vi "Auto.vi"() -> ()   [LabVIEW 2020]
uses:
  Global_Variable/Global.vi
  Global_Variable/A180648.vi
  Global_Variable/System_Conf.vi
  Libraries/S7/S7.lvlib
panel:
  out "前序":string
  out "用户事件输出":refnum<user-event>
  out "磨合正向初始化":bool
  out "工位三开始计时1":bool
  out "产品变更_Event":refnum<user-event>
  out "NVH":bool=TRUE
  out "T1+T2":dbl
  out "T2":dbl
  out "T1":dbl
  out "吸收电流":sgl
  out "输出扭矩(大)":sgl
  out "输入扭矩":sgl
  out "力特性逆向去程":bool
  out "力特性正向去程":bool
  out "力特性逆向回程":bool
  out "力特性正向回程":bool
  out "工位三开始计时":bool
  out "工位二开始计时":bool
  out "功能正向初始化":bool
  out "功能逆向初始化":bool
  out "空载逆向初始化":bool
  out "空载正向初始化":bool
  out "试验项目":T1(tab)
  out "拉力曲线":cluster{dbl[], dbl[]}[](graph)
  out "侧铆曲线":cluster{dbl[], dbl[]}[](graph)
  out "0°曲线":cluster{dbl[], dbl[]}[](graph)
  out "45°曲线":cluster{dbl[], dbl[]}[](graph)
  out "力特性试验":cluster{dbl[], dbl[]}[](graph)
  out "功能试验":cluster{dbl[], dbl[]}[](graph)
  out "电流特性试验":cluster{dbl[], dbl[]}[](graph)
  out "逆向空载试验":cluster{dbl[], dbl[]}[](graph)
  out "磨合":cluster{dbl[], dbl[]}[](graph)
  in  "判定结果":bool[][](array[boolean])=[[TRUE]]
  in  "STEP":string
  # "车速0"
  # "车速1"
  # "车速2"
  # "车速3"
  # "车速4"
  # "车速5"
  # "车速0"
  # "车速1"
  # "车速2"
  # "车速3"
  # "车速4"
  # "车速5"
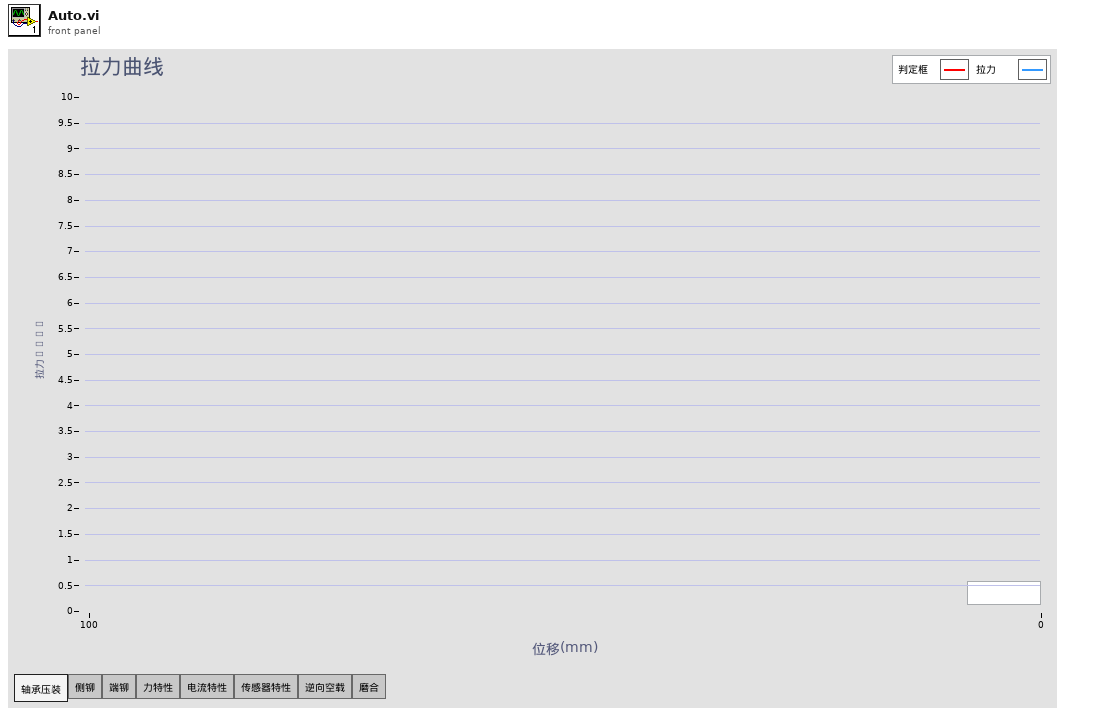
[diagram p1: front panel]
types:
  T1 = enum32{"轴承压装", "侧铆", "端铆", "力特性", "电流特性", "传感器特性", "逆向空载", "磨合"}
  T2 = enum32{"Invalid", "Standard", "Closed", "Hidden", "Minimized", "Maximized"}
  T3 = cluster{"输入轴扭矩":dbl, "输出轴扭矩小量程":dbl, "输出轴扭矩大量程":dbl}
  T4 = typedef "System_conf.ctl" = cluster{"空载滤波":bool, "逆向空载滤波":bool, "空载扭矩系数":dbl, "逆向空载扭矩系数":dbl}
  T5 = cluster{"1位移":cluster{"单位":string, "下限":dbl, "上限":dbl}, "1压力":cluster{"单位":string, "下限":dbl, "上限":dbl}}
  T6 = cluster{"第一段位移区间最大压力":cluster{"单位":string, "下限":dbl, "上限":dbl}, "第一段位移区间最小压力":cluster{"单位":string, "下限":dbl, "上限":dbl}, "压装最终位移":cluster{"单位":string, "下限":dbl, "上限":dbl}}
  T7 = cluster{"卡簧判定结果":cluster{"单位":string, "下限":dbl, "上限":dbl}}
  T8 = typedef "lveventtype.ctl" = enum32{"Null", "Timeout", "Annotation Menu Selection", "Annotation Menu Selection?", "App Instance Close", "App Instance Close?", "Autoscale Range Change", "Bookmark Info Change", "Cell Edit", "Cell Edit?", "Cursor Grab", "Cursor Grab?", "Cursor Menu Selection", "Cursor Menu Selection?", "Cursor Move", "Cursor Release", "Data Change", "Direction Change", "Display State Change", "Drag Ended", "Drag Enter", "Drag Leave", "Drag Over", "Drag Source Update", "Drag Starting", "Drag Starting?", "Drop", "Exec State Change", "Key Down", "Key Down?", "Key Repeat", "Key Repeat?", "Key Up", "Listbox Double Click", "Menu Activation?", "Menu Selection (App)", "Menu Selection? (App)", "Menu Selection (User)", "Mouse Down", "Mouse Down?", "Mouse Enter", "Mouse Leave", "Mouse Move", "Mouse Up", "Mouse Wheel", "NI Security User Change (App)", "Pane Size", "Panel Close", "Panel Close?", "Panel Resize", "Plot Attribute Change", "Scale Range Change", "Shortcut Menu Activation?", "Shortcut Menu Selection (App)", "Shortcut Menu Selection? (App)", "Shortcut Menu Selection (User)", "Tree Double Click", "Tree Drag", "Tree Drag?", "Tree Drop", "Tree Drop?", "Tree Item Close", "Tree Item Close?", "Tree Item Open", "Tree Item Open?", "User Event", "Value Change"}
  T9 = typedef "LVPoint32TypeDef.ctl" = cluster{"Horizontal":i32, "Vertical":i32}
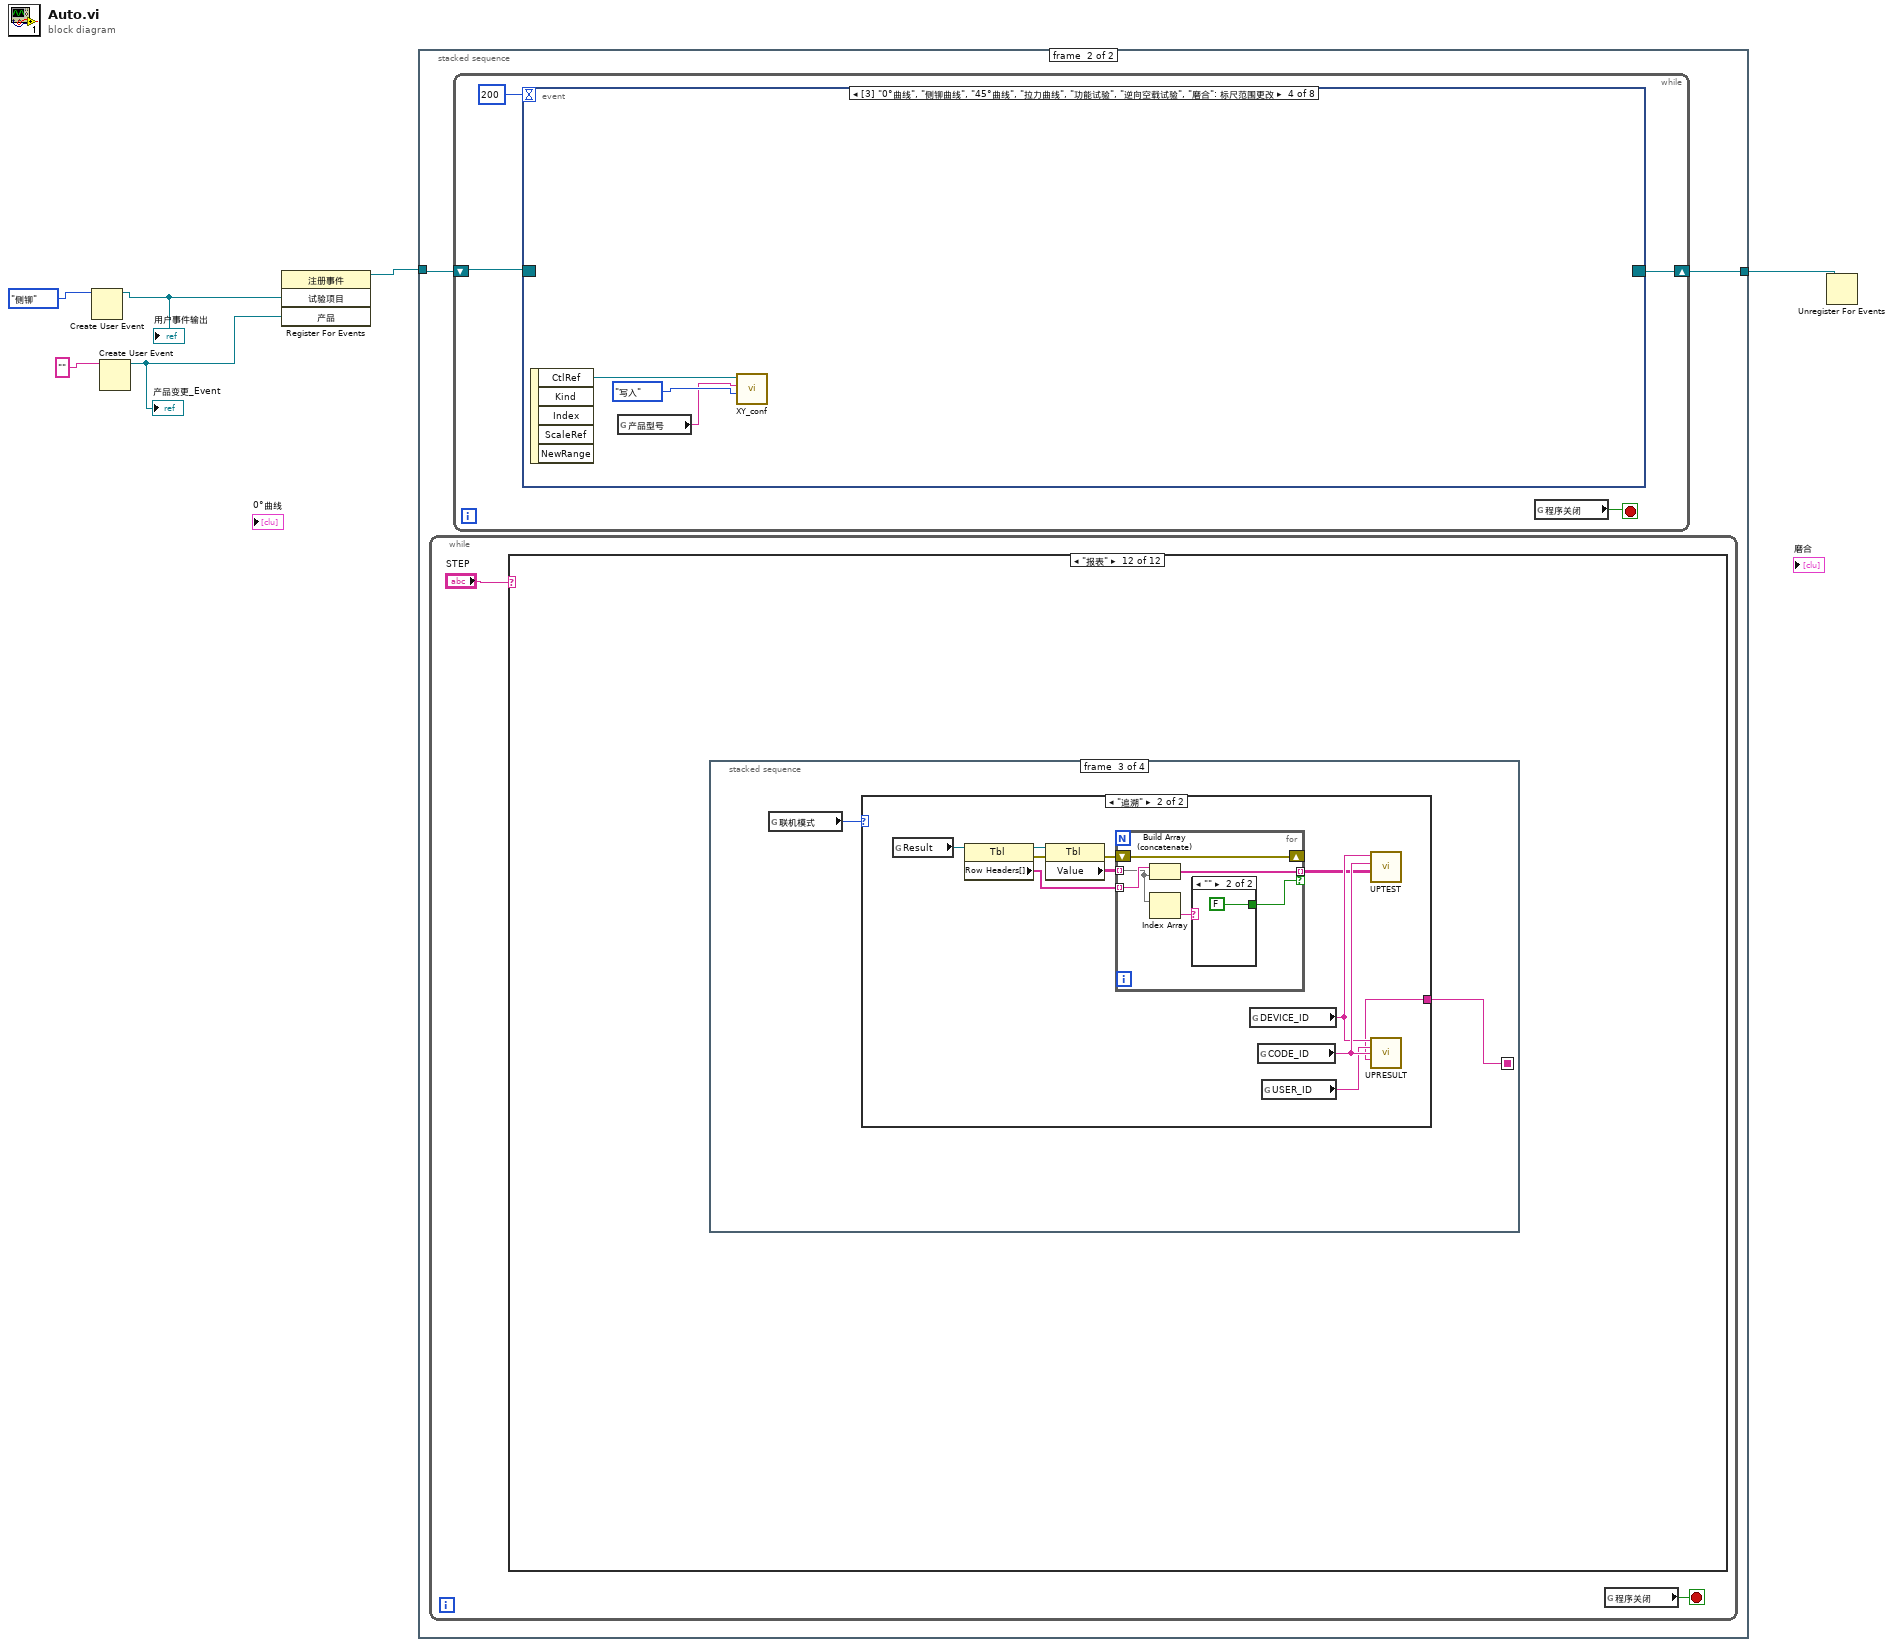
[diagram p0: block diagram]
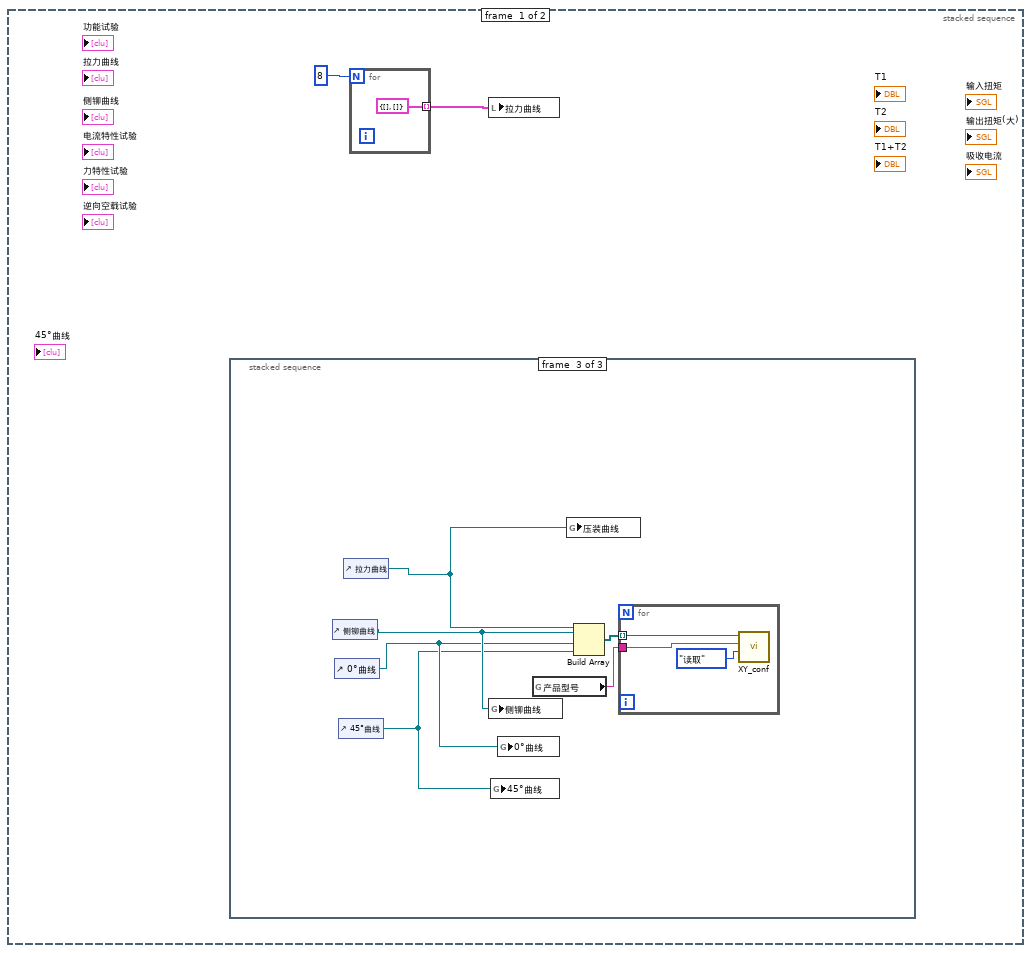
[diagram p2: hidden frame]
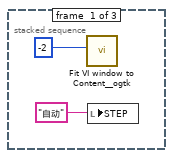
[diagram p3: hidden frame]
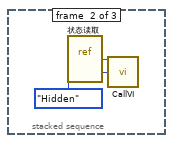
[diagram p4: hidden frame]
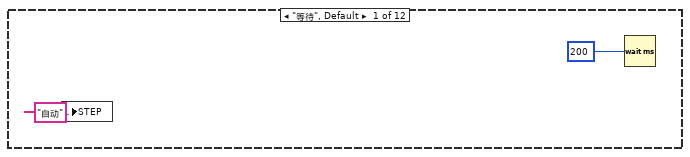
[diagram p5: hidden frame]
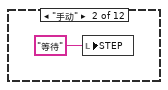
[diagram p6: hidden frame]
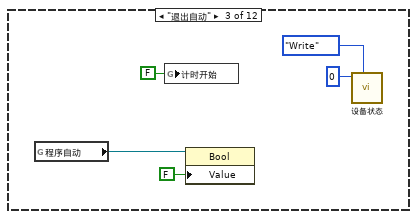
[diagram p7: hidden frame]
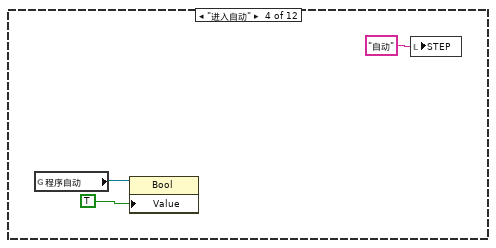
[diagram p8: hidden frame]
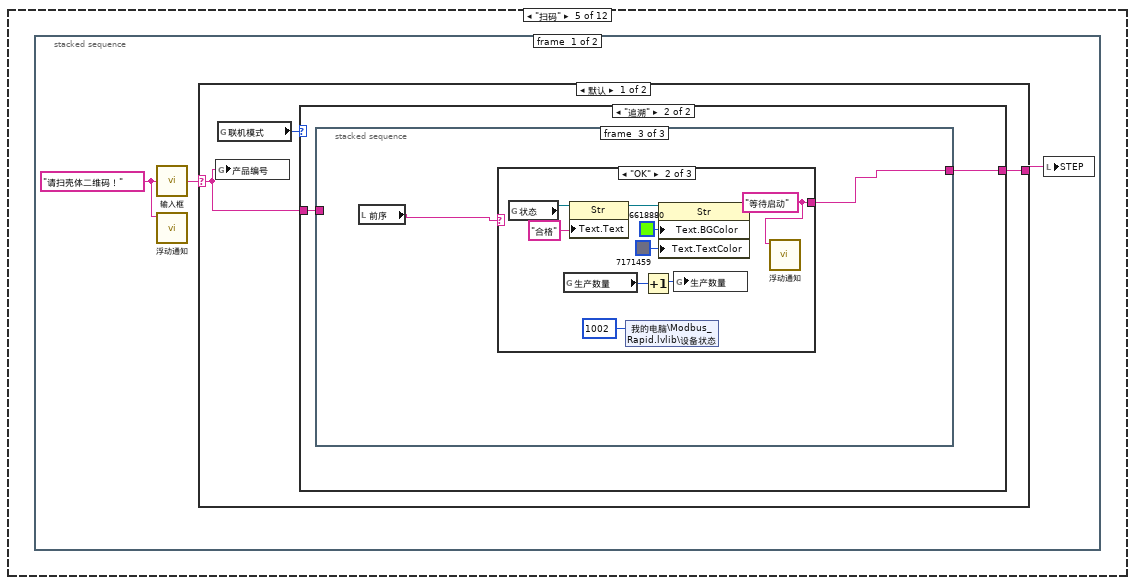
[diagram p9: hidden frame]
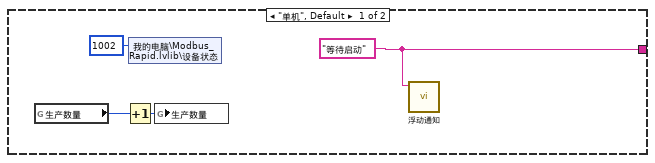
[diagram p10: hidden frame]
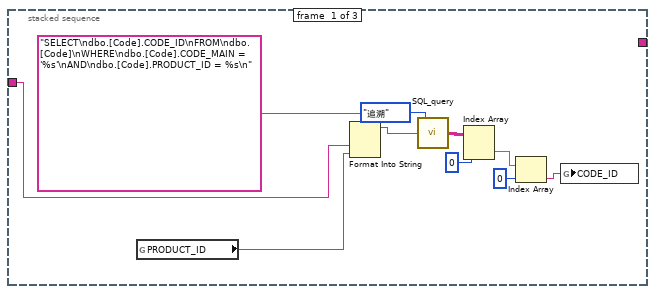
[diagram p11: hidden frame]
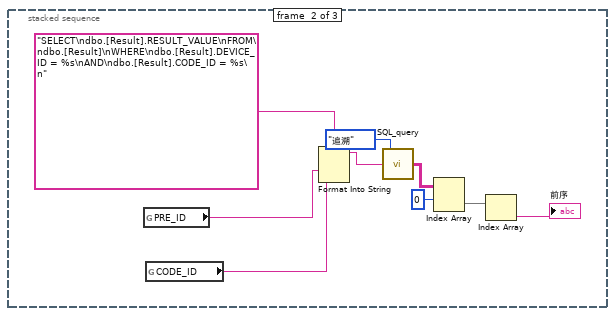
[diagram p12: hidden frame]
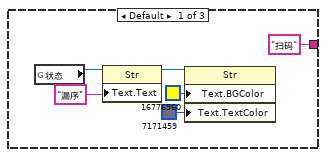
[diagram p13: hidden frame]
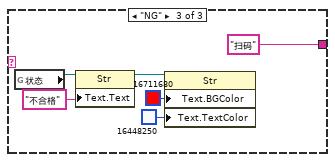
[diagram p14: hidden frame]
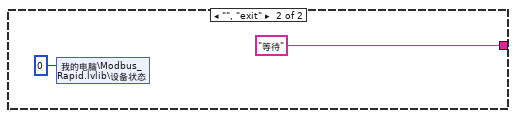
[diagram p15: hidden frame]
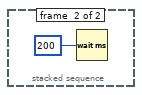
[diagram p16: hidden frame]
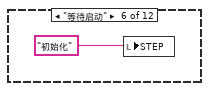
[diagram p17: hidden frame]
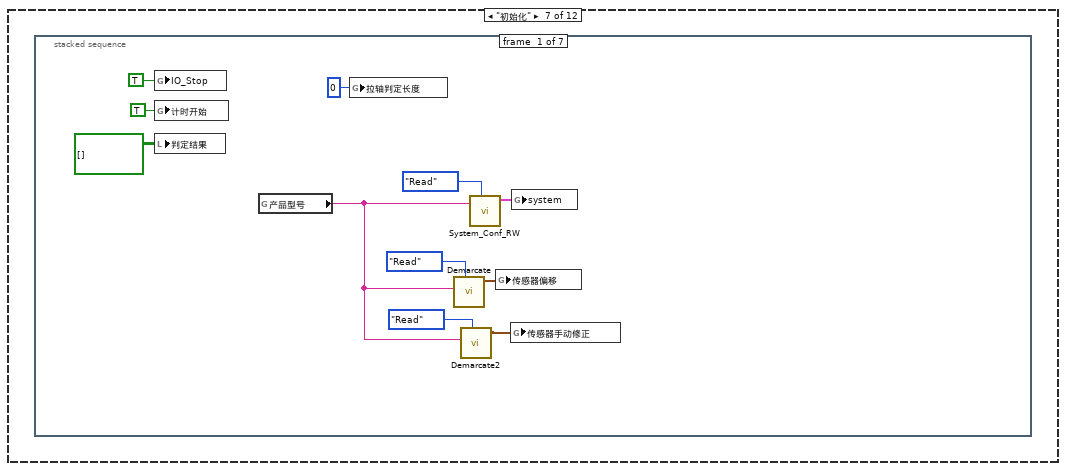
[diagram p18: hidden frame]
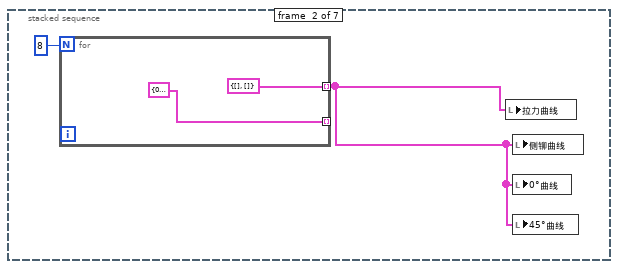
[diagram p19: hidden frame]
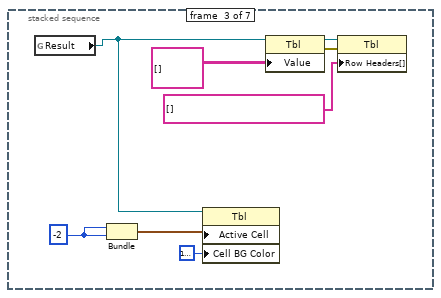
[diagram p20: hidden frame]
diagram:
  n1 = Create User Event(user event datatype=T1."侧铆" ("试验项目")) -> (user event=w1:refnum<user-event>)  [unwired: 1 in, 1 out]
  "用户事件输出" <- w1
  n2 = Create User Event(user event datatype="" ("产品")) -> (user event=w3:refnum<user-event>)  [unwired: 1 in, 1 out]
  "产品变更_Event" <- w3
  n3 = register-events(w1, w3) -> (reference out=w6:refnum<event-registration>)  [unwired: 2 in, 1 out]
  n4 = stacked-sequence {
    tunnel: w6 -> [_ w24]
    tunnel: [_ w23] -> w5
    frame #0 {
      n5 = stacked-sequence {
        frame #0 {
          n6 = call <userlib>:"Fit VI window to Content__ogtk.vi"("border spacing (2 px)"=-2) -> ()  [unwired: 5 in, 2 out]
          n7 = local write "STEP"("自动" ("STEP")) -> ()
        }
        frame #1 {
          n8 = vi-ref "状态读取.vi"() -> (w13:refnum<vi>)
          n9 = call "CallVI.vi"("VI引用"=w13, "状态"=T2."Hidden") -> ()  [unwired: 12 in, 2 out]
        }
        frame #2 {
          n10 = control-ref of="侧铆曲线"() -> (w17:refnum<vi>)
          n11 = control-ref of="0°曲线"() -> (w16:refnum<vi>)
          n12 = control-ref of="45°曲线"() -> (w15:refnum<vi>)
          n13 = control-ref of="拉力曲线"() -> (w14:refnum<vi>)
          n14 = global write "A180648.vi" "侧铆曲线"(w17) -> ()
          n15 = global write "A180648.vi" "45°曲线"(w15) -> ()
          n16 = global write "A180648.vi" "0°曲线"(w16) -> ()
          n17 = global read "Global.vi" "产品型号"() -> (w18:string)
          n18 = global write "A180648.vi" "压装曲线"(w14) -> ()
          n19 = Build Array(w14, w17, w16, w15) -> (w19:refnum<vi>[])
          n20 = for {
            tunnel: w19 -> [w21] mode=indexing
            tunnel: w18 -> [w20]
            n21 = call "XY_conf.vi"("方式"=enum16{"写入", "读取"}."读取", "产品"=w20, "XY图引用"=w21) -> ()  [unwired: 4 in, 1 out]
          }
        }
      }
      n22 = for {
        N: 8 -> [_]
        tunnel: [cluster{dbl[], dbl[]} {[], []}] -> w8 mode=indexing
      }
      n23 = local write "拉力曲线"(w8) -> ()
    }
    frame #1 {
      n24 = while {
        stop <- w26 stop-if-true
        n25 = case shown="\"报表\"" "STEP" {
          frame "等待", Default {
            n26 = local write "STEP"("自动" ("STEP")) -> ()
            n27 = Wait (ms)(milliseconds to wait=u32 200 ("等待时间（毫秒）")) -> ()  [unwired: 1 out]
          }
          frame "手动" {
            n28 = local write "STEP"("等待" ("STEP")) -> ()
          }
          frame "退出自动" {
            n29 = global read "Global.vi" "程序自动"() -> (w31:refnum<vi>)
            n30 = global write "Global.vi" "计时开始"(FALSE ("计时开始")) -> ()
            n31 = property class="Bool"(reference=w31, "Value"=FALSE) -> ()  [unwired: 1 in, 2 out]
            n32 = call "设备状态.vi"("枚举"=enum16{"Read", "Write"}."Write", "Status_Write"=i16 0) -> ()  [unwired: 9 in, 1 out]
          }
          frame "进入自动" {
            n33 = global read "Global.vi" "程序自动"() -> (w36:refnum<vi>)
            n34 = property class="Bool"(reference=w36, "Value"=TRUE) -> ()  [unwired: 1 in, 2 out]
            n35 = local write "STEP"("自动" ("STEP")) -> ()
          }
          frame "扫码" {
            n36 = stacked-sequence {
              frame #0 {
                w39 = "请扫壳体二维码！" ("提示信息")
                n37 = call "输入框.vi"("提示信息"=w39) -> ("条形码输出"=w40:string)
                n38 = call "浮动通知.vi"("通知内容"=w39) -> ()  [unwired: 11 in]
                n39 = case shown="默认" w40 {
                  selector: w40 -> [w41 _]
                  tunnel: [w43 "等待" ("State(s) in Front (\"\")")] -> w38
                  frame Default {
                    n40 = global write "Global.vi" "产品编号"(w41) -> ()
                    n41 = global read "Global.vi" "联机模式"() -> (w42:enum16{"单机", "追溯"})
                    n42 = case shown="\"追溯\"" w42 {
                      tunnel: [w45 w49] -> w43
                      tunnel: w41 -> [_ w48]
                      frame "单机", Default {
                        w45 = "等待启动" ("State(s) in Front (\"\")")
                        n43 = global read "Global.vi" "生产数量"() -> (w46:i32)
                        n44 = Increment(x=w46) -> (x+1=w47:i32)
                        n45 = shared-variable "我的电脑\\Modbus_Rapid.lvlib\\设备状态"(u16 1002 ("设备状态")) -> ()  [unwired: 1 in, 1 out]
                        n46 = global write "Global.vi" "生产数量"(w47) -> ()
                        n47 = call "浮动通知.vi"("通知内容"=w45) -> ()  [unwired: 11 in]
                      }
                      frame "追溯" {
                        n48 = stacked-sequence {
                          tunnel: [_ _ w70] -> w49
                          tunnel: w48 -> [w58 _ _]
                          frame #0 {
                            n49 = global read "追溯Global.vi" "PRODUCT_ID"() -> (w57:string)
                            n50 = Format Into String(format string="SELECT\ndbo.[Code].CODE_ID\nFROM\ndbo.[Code]\nWHERE\ndbo.[Code].CODE_MAIN = '%s'\nAND\ndbo.[Code].PRODUCT_ID = %s\n" ("格式字符串"), w58, w57) -> (resulting string=w56:string)  [unwired: 2 in, 1 out]
                            n51 = call "SQL_query.vi"("SQL query"=w56, "联机模式"=enum16{"单机", "追溯"}."追溯") -> ("data"=w54:string[][])  [unwired: 2 in, 1 out]
                            n52 = Index Array(array=w54, index (row)=0 ("索引 (行)")) -> (element=w52:string[])  [unwired: 1 in]
                            n53 = Index Array(array=w52, index=0 ("索引")) -> (element=w50:string)
                            n54 = global write "追溯Global.vi" "CODE_ID"(w50) -> ()
                          }
                          frame #1 {
                            n55 = global read "追溯Global.vi" "PRE_ID"() -> (w67:string)
                            n56 = global read "追溯Global.vi" "CODE_ID"() -> (w66:string)
                            n57 = Format Into String(format string="SELECT\ndbo.[Result].RESULT_VALUE\nFROM\ndbo.[Result]\nWHERE\ndbo.[Result].DEVICE_ID = %s\nAND\ndbo.[Result].CODE_ID = %s\n" ("格式字符串"), w67, w66) -> (resulting string=w65:string)  [unwired: 2 in, 1 out]
                            n58 = call "SQL_query.vi"("SQL query"=w65, "联机模式"=enum16{"单机", "追溯"}."追溯") -> ("data"=w63:string[][])  [unwired: 2 in, 1 out]
                            n59 = Index Array(array=w63, index (row)=0 ("索引 (行)")) -> (element=w61:string[])  [unwired: 1 in]
                            n60 = Index Array(array=w61) -> (element=→"前序":string)  [unwired: 1 in]
                          }
                          frame #2 {
                            n61 = local read "前序"() -> (w69:string)
                            n62 = case shown="\"OK\"" w69 {
                              tunnel: ["扫码" ("State(s) in Front (\"\")") w80 "扫码" ("State(s) in Front (\"\")")] -> w70
                              frame Default {
                                n63 = global read "Global.vi" "状态"() -> (w76:refnum<vi>)
                                n64 = property class="Str"(reference=w76, "Text.Text"="漏序" ("文本.文本")) -> (reference out=w75:refnum<vi>)  [unwired: 1 in, 1 out]
                                n65 = property class="Str"(reference=w75, "Text.BGColor"=u32 16776960 ("文本.文本颜色:背景色"), "Text.TextColor"=u32 7171459 ("文本.文本颜色:文本颜色")) -> ()  [unwired: 1 in, 2 out]
                              }
                              frame "OK" {
                                w80 = "等待启动" ("State(s) in Front (\"\")")
                                n66 = global read "Global.vi" "状态"() -> (w85:refnum<vi>)
                                n67 = global read "Global.vi" "生产数量"() -> (w78:i32)
                                n68 = property class="Str"(reference=w85, "Text.Text"="合格" ("文本.文本")) -> (reference out=w83:refnum<vi>)  [unwired: 1 in, 1 out]
                                n69 = shared-variable "我的电脑\\Modbus_Rapid.lvlib\\设备状态"(u16 1002 ("设备状态")) -> ()  [unwired: 1 in, 1 out]
                                n70 = Increment(x=w78) -> (x+1=w79:i32)
                                n71 = property class="Str"(reference=w83, "Text.BGColor"=u32 6618880 ("文本.文本颜色:背景色"), "Text.TextColor"=u32 7171459 ("文本.文本颜色:文本颜色")) -> ()  [unwired: 1 in, 2 out]
                                n72 = global write "Global.vi" "生产数量"(w79) -> ()
                                n73 = call "浮动通知.vi"("通知内容"=w80) -> ()  [unwired: 11 in]
                              }
                              frame "NG" {
                                n74 = global read "Global.vi" "状态"() -> (w91:refnum<vi>)
                                n75 = property class="Str"(reference=w91, "Text.Text"="不合格" ("文本.文本")) -> (reference out=w89:refnum<vi>)  [unwired: 1 in, 1 out]
                                n76 = property class="Str"(reference=w89, "Text.BGColor"=u32 16711680 ("文本.文本颜色:背景色"), "Text.TextColor"=u32 16448250 ("文本.文本颜色:文本颜色")) -> ()  [unwired: 1 in, 2 out]
                              }
                            }
                          }
                        }
                      }
                    }
                  }
                  frame "", "exit" {
                    n77 = shared-variable "我的电脑\\Modbus_Rapid.lvlib\\设备状态"(u16 0 ("设备状态")) -> ()  [unwired: 1 in, 1 out]
                  }
                }
                n78 = local write "STEP"(w38) -> ()
              }
              frame #1 {
                n79 = Wait (ms)(milliseconds to wait=u32 200 ("等待时间（毫秒）")) -> ()  [unwired: 1 out]
              }
            }
          }
          frame "等待启动" {
            n80 = local write "STEP"("初始化" ("STEP")) -> ()
          }
          frame "初始化" {
            n81 = stacked-sequence {
              frame #0 {
                n82 = global write "Global.vi" "IO_Stop"(TRUE ("IO_Stop")) -> ()
                n83 = global write "Global.vi" "计时开始"(TRUE ("计时开始")) -> ()
                n84 = local write "判定结果"(bool[][] [] ("判定结果")) -> ()
                n85 = global read "Global.vi" "产品型号"() -> (w97:string)
                n86 = global write "判定参数.vi" "拉轴判定长度"(0 ("拉轴判定长度")) -> ()
                n87 = call "Demarcate.vi"("Mode"=enum16{"Read", "Write"}."Read", "Section"=w97) -> ("Sensor OUT"=w101:T3)  [unwired: 8 in, 1 out]
                n88 = call "Demarcate2.vi"("Mode"=enum16{"Read", "Write"}."Read", "Section"=w97) -> ("Sensor OUT"=w100:T3)  [unwired: 8 in, 1 out]
                n89 = call "System_Conf_RW.vi"("Mode"=enum16{"Read", "Write"}."Read", "Section"=w97) -> ("system_out"=w103:T4)  [unwired: 8 in, 1 out]
                n90 = global write "传感器偏移.vi" "传感器偏移"(w101) -> ()
                n91 = global write "传感器偏移.vi" "传感器手动修正"(w100) -> ()
                n92 = global write "System_Conf.vi" "system"(w103) -> ()
              }
              frame #1 {
                n93 = for {
                  N: 8 -> [_]
                  tunnel: [cluster{dbl[], dbl[]} {[], []}] -> w107 mode=indexing
                  tunnel: [cluster{"f0":dbl, "df":dbl, "magnitude":dbl[]} {"f0"=0.0, "df"=0.0, "magnitude"=[]} ("power spectrum [dB EU]")] -> _ mode=indexing
                }
                n94 = local write "拉力曲线"(w107) -> ()
                n95 = local write "侧铆曲线"(w107) -> ()
                n96 = local write "0°曲线"(w107) -> ()
                n97 = local write "45°曲线"(w107) -> ()
              }
              frame #2 {
                w112 = -2
                n98 = global read "Global.vi" "Result"() -> (w114:refnum<vi>)
                n99 = Bundle(w112, w112) -> (w111:cluster{i32, i32})  [unwired: 1 in]
                n100 = property class="Tbl"(reference=w114, "Active Cell"=w111, "Cell BG Color"=u32 16777216 ("活动单元格:单元格背景色")) -> ()  [unwired: 1 in, 2 out]
                n101 = property class="Tbl"(reference=w114, "Value"=string[][] []) -> (reference out=w117:refnum<vi>, error out=w118:errorcluster)  [unwired: 1 in]
                n102 = property class="Tbl"(reference=w117, error in=w118, "Row Headers[]"=string[] [] ("列首字符串[]")) -> ()  [unwired: 2 out]
              }
              frame #3 {
                n103 = global read "A180648.vi" "LED-轴承压装"() -> (w122:refnum<vi>)
                n104 = global read "A180648.vi" "LED-端铆"() -> (w119:refnum<vi>)
                n105 = global read "A180648.vi" "LED-侧铆"() -> (w120:refnum<vi>)
                n106 = Build Array(w122, w120, w119) -> (w121:refnum<vi>[])
                n107 = for {
                  tunnel: w121 -> [w123] mode=indexing
                  n108 = property class="Bool"(reference=w123, "Colors [4]"=cluster{u32, u32}[] [{12369084, 12369084}] ("颜色[4]")) -> ()  [unwired: 1 in, 2 out]
                }
              }
              frame #4 {
                w126 = 1 ("维数大小")
                n109 = Initialize Array(" " ("字符串"), w126, w126, w126) -> (w128:string[][][])
                n110 = global write "A180648.vi" "当前检测项"(enum32{"拉轴", "卡簧", "完成"}."拉轴" ("当前检测项")) -> ()
                n111 = global write "A180648.vi" "检测结果"(w128) -> ()
              }
              frame #5 {
                n112 = local read "拉力曲线"() -> (w130:cluster{dbl[], dbl[]}[])
                n113 = global read "判定参数.vi" "判定框"() -> (w131:T5)
                n114 = for {
                  tunnel: w130 -> [w134] mode=indexing
                  tunnel: [w133] -> w129 mode=indexing
                  tunnel: w131 -> [w132]
                  i -> [w135]
                  n115 = case shown="0" w135 {
                    tunnel: w134 -> [w136 _]
                    tunnel: [w136 w139] -> w133
                    tunnel: w132 -> [_ w144]
                    frame Default {
                    }
                    frame 0 {
                      n116 = Unbundle By Name(w144) -> ("1位移.下限"=w143:dbl, "1位移.上限"=w142:dbl, "1压力.下限"=w137:dbl, "1压力.上限"=w138:dbl)
                      n117 = Build Array(w142, w142, w143, w143, w142) -> (w141:dbl[])
                      n118 = Build Array(w137, w138, w138, w137, w137) -> (w140:dbl[])
                      n119 = Bundle(w141, w140) -> (w139:cluster{dbl[], dbl[]})  [unwired: 1 in]
                    }
                  }
                }
                n120 = local write "拉力曲线"(w129) -> ()
              }
              frame #6 {
                w146 = TRUE
                n121 = local write "STEP"("试验项" ("STEP")) -> ()
                "工位三开始计时" <- w146
                "工位二开始计时" <- w146
                "空载正向初始化" <- w146
                "空载逆向初始化" <- w146
                "功能正向初始化" <- w146
                "功能逆向初始化" <- w146
                "力特性逆向去程" <- w146
                "力特性正向去程" <- w146
                "力特性逆向回程" <- w146
                "力特性正向回程" <- w146
                "磨合正向初始化" <- w146
                "工位三开始计时1" <- w146
              }
            }
          }
          frame "试验项" {
            n122 = global read "A180648.vi" "当前检测项"() -> (w147:enum32{"拉轴", "卡簧", "完成"})
            n123 = case shown="\"拉轴\", 默认" w147 {
              selector: w147 -> [w149 _]
              tunnel: [w152 "报表" ("STEP")] -> w148
              frame "拉轴", Default {
                n124 = global read "Global.vi" "试验项目"() -> (w150:bool[])
                n125 = Index Array(array=w150, index=w149) -> (element=w151:bool)
                n126 = case shown="真" w151 {
                  tunnel: ["试验项" ("字符串") w159] -> w152
                  tunnel: w149 -> [_ w160]
                  frame False {
                    n127 = global read "A180648.vi" "当前检测项"() -> (w157:enum32{"拉轴", "卡簧", "完成"})
                    n128 = Increment(x=w157) -> (x+1=w156:enum32{"拉轴", "卡簧", "完成"})
                    n129 = global write "A180648.vi" "当前检测项"(w156) -> ()
                    n130 = local read "判定结果"() -> (w153:bool[][])
                    n131 = Build Array (concatenate)(w153, bool[] [FALSE] ("判定结果")) -> (w154:bool[][])
                    n132 = local write "判定结果"(w154) -> ()
                  }
                  frame True {
                    n133 = case shown="\"卡簧\"" w160 {
                      tunnel: ["等待" ("STEP") "等待" ("STEP") "报表" ("STEP")] -> w159
                      frame "拉轴", Default {
                        n134 = call "浮动通知.vi"("通知内容"="拉拔力试验") -> ()  [unwired: 11 in]
                        n135 = property on="试验项目" class="TabCtl (严格)"("Val(Sgnl)"=T1."轴承压装" ("值(信号)")) -> ()  [unwired: 2 in, 2 out]
                      }
                      frame "卡簧" {
                        n136 = call "浮动通知.vi"("通知内容"="卡簧检测") -> ()  [unwired: 11 in]
                      }
                      frame "完成" {
                      }
                    }
                  }
                }
              }
              frame "完成" {
              }
            }
            n137 = local write "STEP"(w148) -> ()
          }
          frame "判定" {
            n138 = stacked-sequence {
              frame #0 {
                n139 = shared-variable "我的电脑\\Modbus_Rapid.lvlib\\设备状态"(u16 0 ("设备状态")) -> ()  [unwired: 1 in, 1 out]
              }
              frame #1 {
                n140 = global read "A180648.vi" "当前检测项"() -> (w169:enum32{"拉轴", "卡簧", "完成"})
                n141 = case shown="\"卡簧\"" w169 {
                  frame "完成", Default {
                  }
                  frame "拉轴" {
                    n142 = global read "判定参数.vi" "拉轴判定参数"() -> (w183:T6)
                    n143 = local read "拉力曲线"() -> (w184:cluster{dbl[], dbl[]}[])
                    n144 = Wait (ms)(milliseconds to wait=u32 150 ("等待时间（毫秒）")) -> ()  [unwired: 1 out]
                    n145 = global read "Global.vi" "Result"() -> (w182:refnum<vi>)
                    n146 = call "压装试验判定.vi"("Result"=w182, "判定参数"=w183, "XY曲线"=w184) -> ("判定项长度"=w173:i32, "OK？"=w172:bool)  [unwired: 7 in]
                    n147 = global read "A180648.vi" "LED-轴承压装"() -> (w178:refnum<vi>)
                    n148 = local read "判定结果"() -> (w174:bool[][])
                    n149 = Select(t=cluster{u32, u32}[] [{6618880, 6618880}, {6618880, 6618880}, {6618880, 6618880}, {6618880, 6618880}] ("颜色[4]"), s=w172, f=cluster{u32, u32}[] [{16711680, 16711680}, {16711680, 16711680}, {16711680, 16711680}, {16711680, 16711680}] ("颜色[4]")) -> (s? t:f=w179:cluster{u32, u32}[])
                    n150 = Build Array(TRUE, w172) -> (w177:bool[])
                    n151 = global write "判定参数.vi" "拉轴判定长度"(w173) -> ()
                    n152 = property class="Bool"(reference=w178, "Colors [4]"=w179) -> ()  [unwired: 1 in, 2 out]
                    n153 = Build Array (concatenate)(w174, w177) -> (w175:bool[][])
                    n154 = case shown="真" w172 {
                      tunnel: ["报表" "试验项"] -> w170
                      frame False {
                        n155 = shared-variable "我的电脑\\Modbus_Rapid.lvlib\\工位1合格状态"(u16 2 ("工位1合格状态")) -> ()  [unwired: 1 in, 1 out]
                      }
                      frame True {
                        n156 = global read "A180648.vi" "当前检测项"() -> (w188:enum32{"拉轴", "卡簧", "完成"})
                        n157 = shared-variable "我的电脑\\Modbus_Rapid.lvlib\\工位1合格状态"(u16 1 ("工位1合格状态")) -> ()  [unwired: 1 in, 1 out]
                        n158 = Increment(x=w188) -> (x+1=w187:enum32{"拉轴", "卡簧", "完成"})
                        n159 = global write "A180648.vi" "当前检测项"(w187) -> ()
                      }
                    }
                    n160 = local write "判定结果"(w175) -> ()
                    n161 = local write "STEP"(w170) -> ()
                  }
                  frame "卡簧" {
                    n162 = global read "判定参数.vi" "卡簧判定参数"() -> (w204:T7)
                    n163 = local read "侧铆曲线"() -> (w205:cluster{dbl[], dbl[]}[])
                    n164 = global read "Global.vi" "Result"() -> (w203:refnum<vi>)
                    n165 = call "侧铆试验判定.vi"("Result"=w203, "判定参数"=w204, "XY曲线"=w205) -> ("判定项长度"=w194:i32, "OK？"=w192:bool)  [unwired: 7 in]
                    n166 = global read "A180648.vi" "LED-侧铆"() -> (w199:refnum<vi>)
                    n167 = local read "判定结果"() -> (w195:bool[][])
                    n168 = Select(t=cluster{u32, u32}[] [{6618880, 6618880}, {6618880, 6618880}, {6618880, 6618880}, {6618880, 6618880}] ("颜色[4]"), s=w192, f=cluster{u32, u32}[] [{16711680, 16711680}, {16711680, 16711680}, {16711680, 16711680}, {16711680, 16711680}] ("颜色[4]")) -> (s? t:f=w200:cluster{u32, u32}[])
                    n169 = Build Array(TRUE, w192) -> (w198:bool[])
                    n170 = global write "判定参数.vi" "卡簧判定长度"(w194) -> ()
                    n171 = property class="Bool"(reference=w199, "Colors [4]"=w200) -> ()  [unwired: 1 in, 2 out]
                    n172 = Build Array (concatenate)(w195, w198) -> (w196:bool[][])
                    n173 = case shown="真" w192 {
                      tunnel: ["报表" "试验项"] -> w191
                      frame False {
                        n174 = shared-variable "我的电脑\\Modbus_Rapid.lvlib\\拍照结果"(u16 2 ("拍照结果")) -> ()  [unwired: 1 in, 1 out]
                      }
                      frame True {
                        n175 = global read "A180648.vi" "当前检测项"() -> (w210:enum32{"拉轴", "卡簧", "完成"})
                        n176 = shared-variable "我的电脑\\Modbus_Rapid.lvlib\\拍照结果"(u16 1 ("拍照结果")) -> ()  [unwired: 1 in, 1 out]
                        n177 = Increment(x=w210) -> (x+1=w209:enum32{"拉轴", "卡簧", "完成"})
                        n178 = global write "A180648.vi" "当前检测项"(w209) -> ()
                      }
                    }
                    n179 = local write "判定结果"(w196) -> ()
                    n180 = local write "STEP"(w191) -> ()
                    "NVH" <- TRUE
                  }
                }
              }
            }
          }
          frame "自动" {
            n181 = global read "Global.vi" "设备状态"() -> (w212:i16)
            n182 = case shown="0" w212 {
              frame -128 {
                n183 = global write "Global.vi" "计时开始"(FALSE ("计时开始")) -> ()
                n184 = call "浮动通知.vi"("通知内容"="复位中……" ("Status")) -> ()  [unwired: 11 in]
              }
              frame Default {
              }
              frame 0 {
                n185 = disable-structure shown="禁用" {
                  frame Disabled {
                    n186 = global write "Global.vi" "计时开始"(FALSE ("计时开始")) -> ()
                  }
                  frame Enabled {
                  }
                }
              }
              frame 1 {
                w216 = 4 ("索引")
                n187 = disable-structure shown="禁用" {
                  frame Disabled {
                    n188 = local read "拉力曲线"() -> (w223:cluster{dbl[], dbl[]}[])
                    n189 = for {
                      tunnel: [w225] -> _ mode=indexing
                      tunnel: w223 -> [w224] mode=indexing
                      i -> [w226]
                      n190 = case shown="2" w226 {
                        tunnel: [_ w227] -> w225
                        tunnel: w224 -> [_ w232]
                        frame Default {
                        }
                        frame 2 {
                          n191 = Unbundle(w232) -> (w231:dbl[], w230:dbl[])
                          n192 = Build Array(w231) -> (w229:dbl[][])  [unwired: 1 in]
                          n193 = Build Array(w230) -> (w228:dbl[][])  [unwired: 1 in]
                          n194 = Bundle(w229, w228) -> (w227:cluster{dbl[][], dbl[][]})  [unwired: 1 in]
                        }
                      }
                    }
                    n195 = local read "拉力曲线"() -> ()  [unwired: 1 in]
                  }
                  frame Enabled {
                  }
                }
                n196 = shared-variable "我的电脑\\Modbus_Rapid.lvlib\\电缸位移"() -> (w220:sgl[])  [unwired: 1 in, 1 out]
                n197 = shared-variable "我的电脑\\Modbus_Rapid.lvlib\\电缸压力"() -> (w218:sgl[])  [unwired: 1 in, 1 out]
                n198 = Index Array(array=w220, index=w216) -> (element=w219:sgl)
                n199 = Index Array(array=w218, index=w216) -> (element=w217:sgl)
                n200 = control-ref of="拉力曲线"() -> (w222:refnum<vi>)
                n201 = call "曲线采集.vi"("曲线引用"=w222, "曲线索引"=1, "X"=w219, "Y"=w217) -> ()  [unwired: 10 in, 2 out]
              }
              frame 2 {
                n202 = local write "STEP"("判定" ("STEP")) -> ()
              }
              frame 5 {
              }
              frame 8 {
                n203 = call "浮动通知.vi"("通知内容"="程序停止！" ("Status")) -> ()  [unwired: 11 in]
              }
              frame 12 {
                n204 = call "浮动通知.vi"("通知内容"="请取记号笔标记！" ("Status")) -> ()  [unwired: 11 in]
              }
              frame 10 {
                n205 = global write "A180648.vi" "当前检测项"(enum32{"拉轴", "卡簧", "完成"}."卡簧" ("当前检测项")) -> ()
                n206 = local write "STEP"("判定" ("STEP")) -> ()
              }
              frame 999 {
                n207 = call "浮动通知.vi"("通知内容"="请启动！" ("Status")) -> ()  [unwired: 11 in]
              }
              frame 1000 {
                n208 = local write "STEP"("扫码" ("STEP")) -> ()
              }
              frame 1002 {
              }
              frame 1024 {
                n209 = local write "STEP"("退出自动" ("STEP")) -> ()
              }
            }
          }
          frame "合格判定" {
            n210 = Wait (ms)(milliseconds to wait=u32 100 ("等待时间（毫秒）")) -> ()  [unwired: 1 out]
            n211 = local write "STEP"("等待" ("STEP")) -> ()
          }
          frame "报表" {
            n212 = stacked-sequence {
              seq-local: [_ w246 _ _] -> [_ _ w251 _]
              frame #0 {
                n213 = global write "Global.vi" "计时开始"(FALSE ("计时开始")) -> ()
                n214 = disable-structure shown="禁用" {
                  frame Disabled {
                    n215 = global read "Global.vi" "产品编号"() -> (w245:string)
                    n216 = call "Get_CODE_ID.vi"("CODE_MAIN"=w245) -> ("CODE_ID"=w244:string)  [unwired: 10 in]
                    n217 = global write "追溯Global.vi" "CODE_ID"(w244) -> ()
                  }
                  frame Enabled {
                  }
                }
              }
              frame #1 {
                n218 = global read "Global.vi" "产品编号"() -> (w247:string)
                n219 = call "Report.vi"("文件重命名"=TRUE, "文件名称"=w247, "检测结果"="判定结果") -> ("PRODUCT_VAULE"=w246:string)  [unwired: 7 in, 1 out]
              }
              frame #2 {
                n220 = global read "Global.vi" "联机模式"() -> (w250:enum16{"单机", "追溯"})
                n221 = case shown="\"追溯\"" w250 {
                  tunnel: w251 -> [_ w252]
                  frame "单机", Default {
                  }
                  frame "追溯" {
                    n222 = global read "Global.vi" "Result"() -> (w254:refnum<vi>)
                    n223 = property class="Tbl"(reference=w254) -> (reference out=w259:refnum<vi>, error out=w256:errorcluster, "Row Headers[]"=w257:string[])  [unwired: 1 in]
                    n224 = property class="Tbl"(reference=w259, error in=w256) -> (error out=w255:errorcluster, "Value"=w258:string[][])  [unwired: 1 out]
                    n225 = for {
                      tunnel: w258 -> [w266] mode=indexing
                      tunnel: w257 -> [w267] mode=indexing
                      tunnel: [w264] -> w253 mode=indexing if=w265
                      shift-right: [w263] -> _
                      shift-left: w255 -> [w263]
                      n226 = Build Array (concatenate)(w267, w266) -> (w264:string[])
                      n227 = Index Array(array=w266) -> (element=w268:string)  [unwired: 1 in]
                      n228 = case shown="\"\"" w268 {
                        tunnel: [TRUE FALSE] -> w265
                        frame Default {
                        }
                        frame "" {
                        }
                      }
                    }
                    n229 = global read "追溯Global.vi" "DEVICE_ID"() -> (w261:string)
                    n230 = global read "追溯Global.vi" "CODE_ID"() -> (w262:string)
                    n231 = global read "追溯Global.vi" "USER_ID"() -> (w260:string)
                    n232 = call "UPTEST.vi"("Result"=w253, "CODE_ID"=w262, "DEVICE_ID"=w261) -> ()  [unwired: 6 in, 1 out]
                    n233 = call "UPRESULT.vi"("DEVICE_ID"=w261, "USER_ID"=w260, "CODE_ID"=w262, "RESULT_VALUE"=w252) -> ()  [unwired: 11 in, 1 out]
                  }
                }
              }
              frame #3 {
                n234 = global read "检测结果.vi" "合格状态"() -> (w272:string)
                n235 = local write "STEP"("自动" ("STEP")) -> ()
                n236 = shared-variable "我的电脑\\Modbus_Rapid.lvlib\\设备状态"(u16 1000 ("设备状态")) -> ()  [unwired: 1 in, 1 out]
                n237 = case shown="\"合格\"" w272 {
                  frame "假", Default {
                  }
                  frame "合格" {
                    n238 = global read "Global.vi" "合格数量"() -> (w275:i32)
                    n239 = Increment(x=w275) -> (x+1=w274:i32)
                    n240 = global write "Global.vi" "合格数量"(w274) -> ()
                  }
                }
              }
            }
          }
        }
        n241 = global read "Global.vi" "程序关闭"() -> (w26:bool)
      }
      n242 = while {
        shift-right: [w276] -> w23
        shift-left: w24 -> [w277]
        stop <- w278 stop-if-true
        n243 = event shown="[3] \"0°曲线\", \"侧铆曲线\", \"45°曲线\", \"拉力曲线\", \"功能试验\", \"逆向空载试验\", \"磨合\": 标尺范围更改" {
          selector: w277 -> [_ _ _ _ _ _ _ _]
          dyn-events: [_ _ _ _ _ _ _ _] -> w276
          timeout: 200 -> [_ _ _ _ _ _ _ _]
          event Timeout {
            n244 = event-data() -> ()  [unwired: 1 in, 3 out]
            n245 = call "Obtain Broadcast Events for Registration.vi"() -> ("Already running?"=w280:bool)  [unwired: 9 in, 2 out]
            n246 = case shown="真" w280 {
              frame False {
                n247 = local write "STEP"("手动" ("STEP")) -> ()
              }
              frame True {
                n248 = call "错误代码.vi"() -> ("Status_Read"=w282:u32)  [unwired: 11 in]
                n249 = feedback #1() -> (w292:u32)  [unwired: 1 in]
                n250 = feedback-in #1(w282) -> ()
                n251 = case shown="0" w282 {
                  frame 0 {
                    n252 = global read "Global.vi" "报警图标"() -> (w293:refnum<vi>)
                    n253 = property class="Bool"(reference=w293, "Visible"=FALSE ("可见")) -> ()  [unwired: 1 in, 2 out]
                  }
                  frame 1, Default {
                    n254 = global read "Global.vi" "报警图标"() -> (w296:refnum<vi>)
                    n255 = property class="Bool"(reference=w296, "Visible"=TRUE ("可见")) -> ()  [unwired: 1 in, 2 out]
                  }
                }
                n256 = Greater Or Equal?(x=w282, y=i16 5000) -> (x >= y?=w290:bool)
                n257 = Less?(x=w282, y=i16 5200) -> (x < y?=w291:bool)
                n258 = Equal?(x=w282, y=w292) -> (x = y?=w289:bool)
                n259 = global read "Global.vi" "报警图标"() -> (w284:refnum<vi>)
                n260 = And(x=w290, y=w291) -> (x .and. y?=w283:bool)
                n261 = property class="Bool"(reference=w284, "Value"=w283) -> ()  [unwired: 1 in, 2 out]
                n262 = Bundle By Name(cluster=errorcluster {"status"=FALSE, "code"=0, "source"=""} ("错误常量"), "status"=w283, "code"=w282) -> (w288:errorcluster)
                n263 = case shown="假" w289 {
                  tunnel: w288 -> [w297 _]
                  frame False {
                    n264 = call "报警处理.vi"("错误常量"=w297) -> ()  [unwired: 9 in, 2 out]
                  }
                  frame True {
                  }
                }
              }
            }
          }
          event User Event {
            n265 = event-data() -> ("试验项目"=w298:T1)  [unwired: 1 in]
            "试验项目" <- w298
            n266 = disable-structure shown="禁用" {
              disable-tunnel: w298 -> [w299 _]
              frame Disabled {
                n267 = global read "A180648.vi" "检测结果"() -> (w302:string[][][])
                n268 = global read "Global.vi" "Result"() -> (w300:refnum<vi>)
                n269 = Index Array(array=w302, index (dim 0)=w299) -> (element=w301:string[][])  [unwired: 2 in]
                n270 = property class="Tbl"(reference=w300, "Value"=w301) -> ()  [unwired: 1 in, 2 out]
              }
              frame Enabled {
              }
            }
          }
          event "试验项目": Value Change {
            n271 = event-data() -> ("NewVal"=w303:T1)  [unwired: 1 in]
            n272 = disable-structure shown="禁用" {
              disable-tunnel: w303 -> [w307 _]
              frame Disabled {
                n273 = global read "A180648.vi" "检测结果"() -> (w306:string[][][])
                n274 = global read "Global.vi" "Result"() -> (w304:refnum<vi>)
                n275 = Index Array(array=w306, index (dim 0)=w307) -> (element=w305:string[][])  [unwired: 2 in]
                n276 = property class="Tbl"(reference=w304, "Value"=w305) -> ()  [unwired: 1 in, 2 out]
              }
              frame Enabled {
              }
            }
          }
          event "0°曲线", "侧铆曲线", "45°曲线", "拉力曲线", "功能试验", "逆向空载试验", "磨合": Scale Range Change {
            n277 = event-data() -> ("CtlRef"=w309:refnum<vi>)  [unwired: 1 in, 4 out]
            n278 = global read "Global.vi" "产品型号"() -> (w308:string)
            n279 = call "XY_conf.vi"("方式"=enum16{"写入", "读取"}."写入", "产品"=w308, "XY图引用"=w309) -> ()  [unwired: 4 in, 1 out]
          }
          event User Event {
            n280 = event-data() -> ("产品"=w313:string)  [unwired: 1 in]
            n281 = control-ref of="0°曲线"() -> (w312:refnum<vi>)
            n282 = control-ref of="拉力曲线"() -> (w315:refnum<vi>)
            n283 = control-ref of="45°曲线"() -> (w311:refnum<vi>)
            n284 = control-ref of="侧铆曲线"() -> (w317:refnum<vi>)
            n285 = control-ref of="力特性试验"() -> (w316:refnum<vi>)
            n286 = Build Array(w312, w315, w311, w317, w316) -> (w314:refnum<vi>[])
            n287 = for {
              tunnel: w314 -> [w319] mode=indexing
              tunnel: w313 -> [w318]
              n288 = call "XY_conf.vi"("方式"=enum16{"写入", "读取"}."读取", "产品"=w318, "XY图引用"=w319) -> ()  [unwired: 4 in, 1 out]
            }
          }
          event Panel Close {
            n289 = event-data() -> ()  [unwired: 1 in, 4 out]
            n290 = global write "Global.vi" "程序关闭"(TRUE ("程序关闭")) -> ()
          }
          event "0°曲线", "侧铆曲线", "45°曲线", "拉力曲线", "功能试验", "逆向空载试验", "磨合": Mouse Enter; "0°曲线", "侧铆曲线", "45°曲线", "拉力曲线", "功能试验", "逆向空载试验", "磨合": Mouse Leave; "0°曲线", "侧铆曲线", "45°曲线", "拉力曲线", "功能试验", "逆向空载试验": Cursor Move; "磨合": Mouse Move {
            n291 = event-data() -> ("CtlRef"=w324:refnum<vi>, "Type"=w322:T8)  [unwired: 1 in]
            n292 = call "CursorShow.vi"("nameShow"=TRUE, "Type"=w322, "Graph"=w324) -> ()  [unwired: 7 in, 2 out]
          }
          event "0°曲线", "侧铆曲线", "45°曲线", "拉力曲线", "功能试验", "逆向空载试验", "磨合": Mouse Down {
            n293 = event-data() -> ("CtlRef"=w329:refnum<vi>, "Coords"=w328:T9, "Type"=w326:T8)  [unwired: 1 in]
            n294 = invoke class="XYGraph (严格)" method="Map Coords To XY"(reference=w329, "Coords"=w328) -> (reference out=w327:refnum<vi>, "XY"=w325:cluster{"X":dbl, "Y":dbl})  [unwired: 5 in, 5 out]
            n295 = call "CursorShow.vi"("游标.游标位置"=w325, "Type"=w326, "Graph"=w327) -> ()  [unwired: 7 in, 2 out]
          }
        }
        n296 = global read "Global.vi" "程序关闭"() -> (w278:bool)
      }
    }
  }
  n297 = Unregister For Events(event registration refnum=w5) -> ()  [unwired: 1 in, 1 out]
